vi "Sensor de Flujo_hego.vi"() -> ()   [LabVIEW 2015]
uses:
  <vilib>/LabVIEW Interface for Arduino/Type Defs/Connection Type.ctl
  <vilib>/LabVIEW Interface for Arduino/Type Defs/Board Type.ctl
  <vilib>/LabVIEW Interface for Arduino/Type Defs/Pin Mode.ctl
  <vilib>/LabVIEW Interface for Arduino/LabVIEW Interface for Arduino.lvlib
  <vilib>/ptbypt/NI_PtbyPt.lvlib
panel:
  in  "Digital I/O Pin (0)":u8
  in  "VISA resource":refnum<visa-resource-name>
  out "LITROS POR MINUTO":dbl(graph)
  out "Horizontal Graduated Bar":dbl(slide) scale=0.0..100.0
  out "LITROS POR MINUTO 2":dbl(knob) scale=0.0..100.0
  out "Numeric":i32
  out "PULSOS POR SEGUNDO":i32
  out "CONTRO TIEMPO":dbl
  out "CONTEO":i32
  out "?":bool
  out "LITROS POR MINUTO":dbl
  out "?":string
  out "?":bool
  in  "?":bool
  # "MEDICIÓN DE FLUJO ATRAVEZ DEL SENSOR YF-S201"
  # "Militros/min"
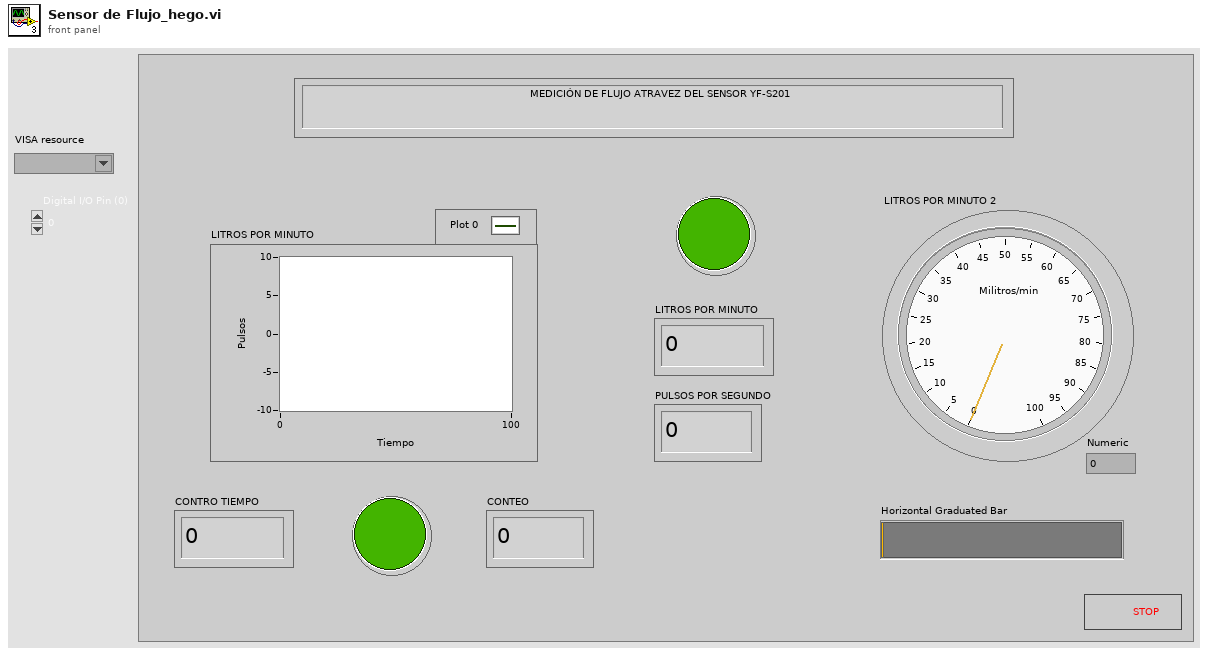
[diagram p1: front panel]
types:
  T1 = typedef "LabVIEW Interface for Arduino.lvlib/Board Type.ctl" = enum16{"Uno", "Dimuelanove w/Atmega 328", "Mega 2560"}
  T2 = typedef "LabVIEW Interface for Arduino.lvlib/Connection Type.ctl" = enum8{"USB / Serial", "XBEE", "BlueSmirf (Bluetooth)"}
  T3 = typedef "LabVIEW Interface for Arduino.lvlib/Arduino Resource.ctl" = cluster{"VISA resource":refnum<visa-resource-name>, "Board Type":T1, "Connection Type":enum8{"USB / Serial"}, "Bytes Per Packet (15)":u8}
  T4 = typedef "LabVIEW Interface for Arduino.lvlib/Pin Mode.ctl" = enum8{"Input", "Output"}
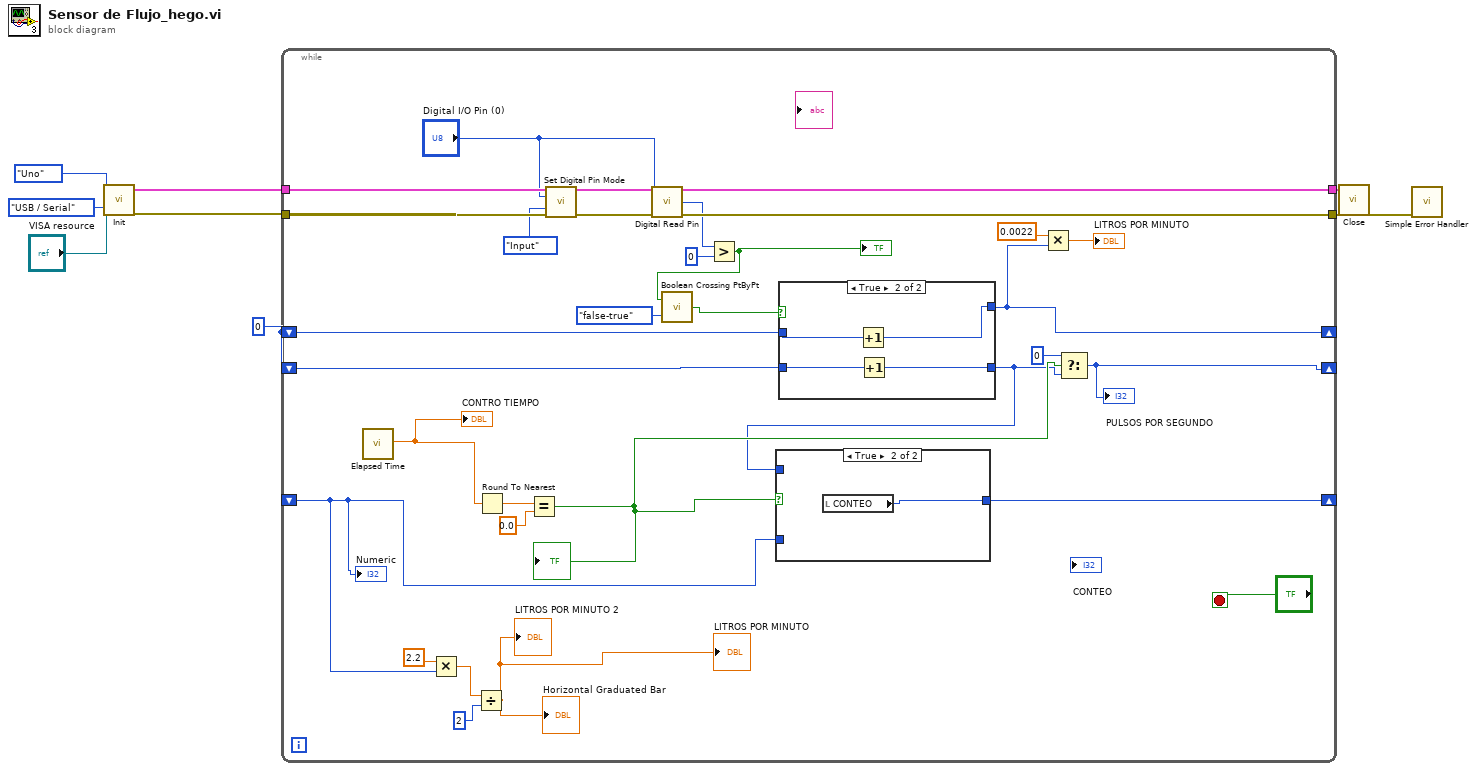
[diagram p0: block diagram]
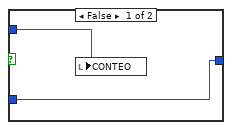
[diagram p2: hidden frame]
diagram:
  w2 = 0 ("CONTADOR 2")
  n1 = call <vilib>:"Init.vi"("VISA resource"="VISA resource", "Board Type (Uno)"=Board_Type."Uno", "Connection Type (USB/Serial)"=Connection_Type."USB / Serial") -> ("Arduino Resource"=w9:T3, "error out"=w8:errorcluster)  [unwired: 15 in]
  n2 = while {
    tunnel: w9 -> [w41]
    tunnel: w8 -> [w40]
    tunnel: [w33] -> w7
    tunnel: [w32] -> w5
    shift-right: [w29] -> _
    shift-left: w2 -> [w28]
    shift-right: [w19] -> _
    shift-left: w2 -> [w23]
    shift-right: [w18] -> _
    shift-left: _ -> [w15]
    stop <- "?" stop-if-true
    n3 = call "Elapsed Time"() -> ("Elapsed Time (s)"=w13:dbl)  [unwired: 12 in, 7 out]
    "CONTRO TIEMPO" <- w13
    n4 = Multiply(x=2.2, y=w15) -> (x*y=w14:dbl)
    n5 = Divide(x=w14, y=2) -> (x/y=→"LITROS POR MINUTO 2" →"Horizontal Graduated Bar" →"LITROS POR MINUTO":dbl)
    n6 = Round To Nearest(number=w13) -> (nearest integer value=w12:dbl)
    n7 = Equal?(x=w12, y=0.0) -> (x = y?=w21:bool)
    "?" <- w21
    n8 = call <vilib>:"Set Digital Pin Mode.vi"("Arduino Resource"=w41, "Digital I/O Pin"="Digital I/O Pin (0)", "Pin Mode (Input)"=Pin_Mode."Input", "error in"=w40) -> ("Arduino Resource"=w37:T3, "error out"=w36:errorcluster)  [unwired: 10 in]
    n9 = call <vilib>:"Digital Read Pin.vi"("Arduino Resource"=w37, "Digital I/O Pin (0)"="Digital I/O Pin (0)", "error in"=w36) -> ("Arduino Resource"=w33:T3, "Value"=w31:u8, "error out"=w32:errorcluster)  [unwired: 10 in]
    n10 = Greater?(x=w31, y=0) -> (0:w26:bool)
    "?" <- w26
    n11 = call <vilib>:"Boolean Crossing PtByPt.vi"("direction"=enum16{"either", "false-true", "true-false"}."false-true", "input"=w26) -> ("crossing"=w25:bool)  [unwired: 1 in]
    n12 = case shown="True" w25 {
      tunnel: [w46 w50] -> w29
      tunnel: w28 -> [w46 w49]
      tunnel: w23 -> [w45 w48]
      tunnel: [w45 w47] -> w20
      frame False {
      }
      frame True {
        n13 = Increment(x=w49) -> (x+1=w50:i32)
        n14 = Increment(x=w48) -> (x+1=w47:i32)
      }
    }
    n15 = case shown="True" w21 {
      tunnel: w20 -> [w43 _]
      tunnel: [w42 w44] -> w18
      tunnel: w15 -> [w42 _]
      frame False {
        n16 = local write "CONTEO"(w43) -> ()
      }
      frame True {
        n17 = local read "CONTEO"() -> (w44:i32)
      }
    }
    n18 = Multiply(x=0.0022, y=w29) -> (x*y=→"LITROS POR MINUTO":dbl)
    n19 = Select(t=0, s=w21, f=w20) -> (s? t:f=w19:i32)
    "PULSOS POR SEGUNDO" <- w19
    "Numeric" <- w15
  }
  n20 = call <vilib>:"Close.vi"("Arduino Resource"=w7, "error in"=w5) -> ("error out"=w6:errorcluster)  [unwired: 13 in]
  n21 = call <vilib>:"Simple Error Handler.vi"("error in (no error)"=w6) -> ()  [unwired: 4 in, 5 out]
